vi "Configure Serial Stream.vi"(7 "Mode (Raw)":T5, 8 "error in (no error)":errorcluster, 10 "Port Config (115200 8N1)":T1={"Baud (115200)"=115200, "Data Bits (8)"=8, "Stop Bits (1)"=10, "Flow Control"=0, "LineTerm (\\n)"="\n", "Timeout ms (10000)"=10000, "Parity (None)"=enum."None"} {"Flow Control" items=["None", "XON/XOFF", "RTS/CTS", "XON/XOFF & RTS/CTS", "DTR/DSR", "XON/XOFF & DTR/DSR"]; "Stop Bits (1)" items=["1.0"=10, "1.5"=15, "2.0"=20]}, 11 "Serial Port":refnum<visa-resource-name>) -> (0 "error out":errorcluster, 3 "Serial Client out":refnum<class "Serial Client.lvclass">)   [LabVIEW 2020, in "Stream-Serial.lvlib" / "Serial Client.lvclass"]
doc: "Initializes a new Serial Client instance with the specified communication mode and port configuration. Note that the LineTerm config (defaults to \\n) only applies when the Mode is set to LineTerm. This is a convenience method instead of separately calling the Ctor VI, setting the resource as a string, and configuring the port parameters.\n\n<b>Mode</b> has the following values:\n - <b>Raw</b> - Reads and writes the exact number of bytes specified. If the number of bytes in a read aren't available by <b>Timeout</b> then the read will timeout and the number of bytes that were able to be read will be returned. No extra bytes are added or stripped with data transferred. This is the likely mode when communicating with an instrument or device that uses binary data.\n\n- <b>Buffered</b> - Data is transferred as complete packets and the length of each packet is prepended (4 bytes) to the packet transferred. When reading, the number of bytes input is ignored and an entire packet is returned or the read will timeout if a full packet is not available. This mode is intended to be used with another <b>Serial Client</b> controlling the remote port but can also be useful with other devices and software that follows this same mechanism and can mix binary and ascii data.\n\n- <b>LineTerm</b> - Intended for line-based ASCII communication and is used with nearly all instruments and devices that transfer data in ASCII. Similar to <b>Buffered</b> mode when reading data an entire line will be returned or if a line termination hasn't been found then the read will timeout."
uses:
  Serial Client.lvclass
  C:/Program Files (x86)/National Instruments/LabVIEW 2020/vi.lib/IlluminatedG/lv-stream/Endpoint/Endpoint.lvclass
  <vilib>/IlluminatedG/lv-stream/stream/Mode.ctl
  Port Config.ctl
  Stop Bits.ctl
  Flow Control.ctl
  Parity.ctl
  Serial Client.lvclass/Serial Client.ctl
  <vilib>/IlluminatedG/lv-stream/Endpoint/Endpoint.lvclass
  <vilib>/IlluminatedG/lv-stream/Stream.lvlib
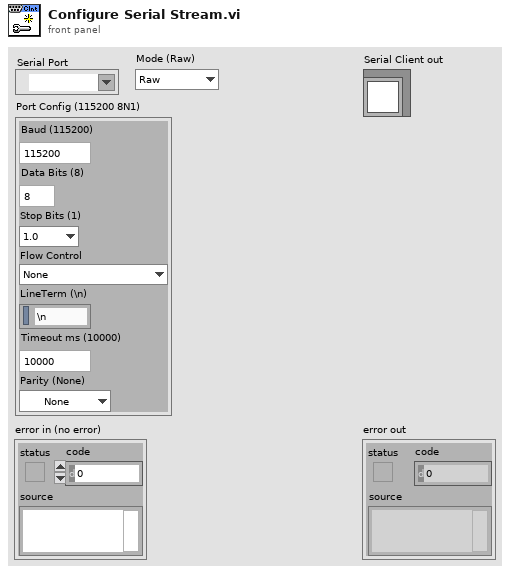
[diagram p1: front panel]
types:
  T1 = typedef "Stream-Serial.lvlib/Serial Client.lvclass/Port Config.ctl" = cluster{"Baud (115200)":u32, "Data Bits (8)":u8, "Stop Bits (1)":T2, "Flow Control":T3, "LineTerm (\\n)":string, "Timeout ms (10000)":i32, "Parity (None)":T4}
  T2 = typedef "Stream-Serial.lvlib/Serial Client.lvclass/Stop Bits.ctl" = u16
  T3 = typedef "Stream-Serial.lvlib/Serial Client.lvclass/Flow Control.ctl" = u16
  T4 = typedef "Stream-Serial.lvlib/Serial Client.lvclass/Parity.ctl" = enum16{"None", "Odd", "Even", "Mark", "Space"}
  T5 = typedef "Stream.lvlib/Mode.ctl" = enum16{"Raw", "Buffered", "LineTerm"}
  T6 = typedef "Stream-Serial.lvlib/Serial Client.lvclass/Ref Data.ctl" = cluster{"Stream":refnum<class "Serial Stream.lvclass">, "State":T7, "Client Loop":refnum<vi>, "Port Config":T1, "VISA Resource":refnum<visa-resource-name>}
  T7 = typedef "Stream-Serial.lvlib/Serial Client.lvclass/Connection State.ctl" = enum16{"Closed", "Idle", "Connecting", "Connected", "Shutdown"}
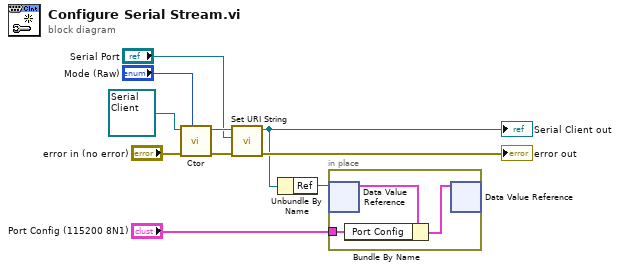
[diagram p0: block diagram]
diagram:
  n1 = call-dynamic "Ctor.vi"("Mode (Raw)"="Mode (Raw)", "error in (no error)"="error in (no error)", "VISA Client in"=refnum<class "Serial Client.lvclass"> refnum) -> ("error out"=w6:errorcluster, "VISA Client out"=w7:refnum<class "Serial Client.lvclass">)  [unwired: 7 in]
  n2 = call <vilib>:"Set URI String.vi"("error in (no error)"=w6, "URI String"="Serial Port", "Endpoint in"=w7) -> ("error out"=→"error out":errorcluster, "Endpoint out"=w1:refnum<class "Serial Client.lvclass">)  [unwired: 7 in]
  "Serial Client out" <- w1
  n3 = Unbundle By Name(w1) -> ("Ref"=w4:refnum<data-value>)
  n4 = in-place {
    in-place-border: "Port Config (115200 8N1)" -> [w11]
    n5 = in-place-dvr #1(w4) -> (w13:T6)  [unwired: 1 out]
    n6 = Bundle By Name(cluster=w13, "Port Config"=w11) -> (w12:T6)
    n7 = in-place-dvr #1(w12) -> ()  [unwired: 2 out]
  }
